vi "subDCRConnect.vi"() -> (0 "Firmware Version":string, 1 "VISA resource name Out":refnum<visa-resource-name>="COM7", 2 "ConnectStatus":bool)   [LabVIEW 2012]
uses:
  <vilib>/Instr/_visa.llb/VISA Configure Serial Port (Instr).vi
panel:
  in  "VISA resource name":refnum<visa-resource-name>="COM2"
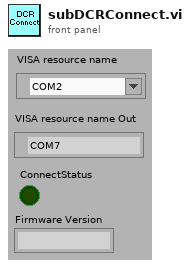
[diagram p1: front panel]
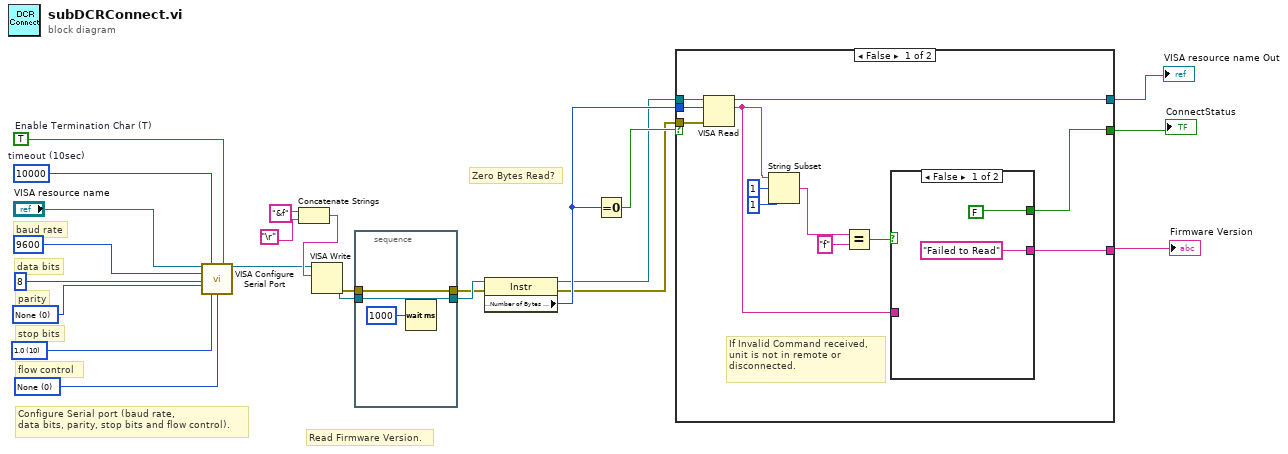
[diagram p0: block diagram]
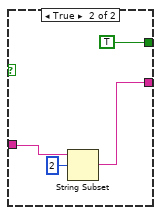
[diagram p2: hidden frame]
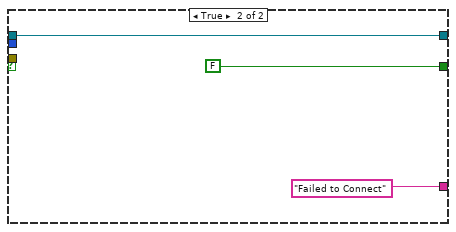
[diagram p3: hidden frame]
diagram:
  w15 = u16 0 items=["None"=0, "XON/XOFF"=1, "RTS/CTS"=2, "DTR/DSR"=4] ("flow control")
  w16 = u16 10 items=["1.0"=10, "1.5"=15, "2.0"=20] ("stop bits")
  w17 = u16 0 items=["None", "Odd", "Even", "Mark", "Space"] ("parity")
  w20 = TRUE  # Enable Termination Char (T)
  w21 = u32 10000  # timeout (10sec)
  # "Zero Bytes Read?"
  # "Read Firmware Version."
  # "flow control"
  # "stop bits"
  # "parity"
  # "data bits"
  # "baud rate"
  # "Configure Serial port (baud rate,\ndata bits, parity, stop bits and flow control)."
  n1 = call-poly "VISA Configure Serial Port"("VISA resource name"="VISA resource name", "timeout (10sec)"=w21, "Enable Termination\nChar (T)"=w20, "baud rate (9600)"=u32 9600 ("baud rate"), "data bits (8)"=u16 8 ("data bits"), "parity (0:none)"=w17, "stop bits (10: 1 bit)"=w16, "flow control (0:none)"=w15) -> ("VISA resource name out"=w4:refnum<visa-resource-name>)  [unwired: 1 in, 6 out]
  n2 = Concatenate Strings("&f" ("write buffer"), "\r") -> (w11:string)
  n3 = VISA Write(VISA resource name=w4, write buffer=w11) -> (VISA resource name out=w14:refnum<visa-resource-name>, error out=w9:errorcluster)  [unwired: 1 in, 1 out]
  n4 = stacked-sequence {
    tunnel: w9 -> [w25]
    tunnel: [w25] -> w10
    tunnel: [w24] -> _
    tunnel: w14 -> [w24]
    frame #0 {
      n5 = Wait (ms)(milliseconds to wait=u32 1000) -> ()  [unwired: 1 out]
    }
  }
  n6 = property class="Instr"(reference=w14, error in=w10) -> (reference out=w5:refnum<visa-resource-name>, error out=w6:errorcluster, "Serial Settings:Number of Bytes at Serial Port"=w7:u32)
  n7 = Equal To 0?(x=w7) -> (x = 0?=w8:bool)
  n8 = case shown="False" w8 {
    tunnel: [w26 FALSE] -> w2
    tunnel: w7 -> [w36 _]
    tunnel: w6 -> [w35 _]
    tunnel: [w34 w45] -> w1
    tunnel: w5 -> [w37 w45]
    tunnel: [w29 "Failed to Connect"] -> w3
    frame False {
      # "If Invalid Command received,\nunit is not in remote or\ndisconnected."
      n9 = VISA Read(VISA resource name=w37, byte count=w36, error in (no error)=w35) -> (VISA resource name out=w34:refnum<visa-resource-name>, read buffer=w27:string)  [unwired: 2 out]
      n10 = String Subset(string=w27, offset (0)=1, length (rest)=1 ("length (rest)")) -> (substring=w28:string)
      n11 = Equal?(x=w28, y="f") -> (x = y?=w30:bool)
      n12 = case shown="False" w30 {
        tunnel: ["Failed to Read" w40] -> w29
        tunnel: w27 -> [_ w41]
        tunnel: [FALSE TRUE] -> w26
        frame False {
        }
        frame True {
          n13 = String Subset(string=w41, offset (0)=2) -> (substring=w40:string)  [unwired: 1 out]
        }
      }
    }
    frame True {
    }
  }
  "VISA resource name Out" <- w1
  "Firmware Version" <- w3
  "ConnectStatus" <- w2
